vi "读取产品参数信息-CCDA.vi"(8 "错误输入（无错误）":errorcluster, 11 "LoadProductName":string) -> (0 "错误输出":errorcluster)   [LabVIEW 2017]
uses:
  Global System.vi
panel:
  in  "名称或相对路径 2":string="BlackTemplete"
  out "连接的字符串":string
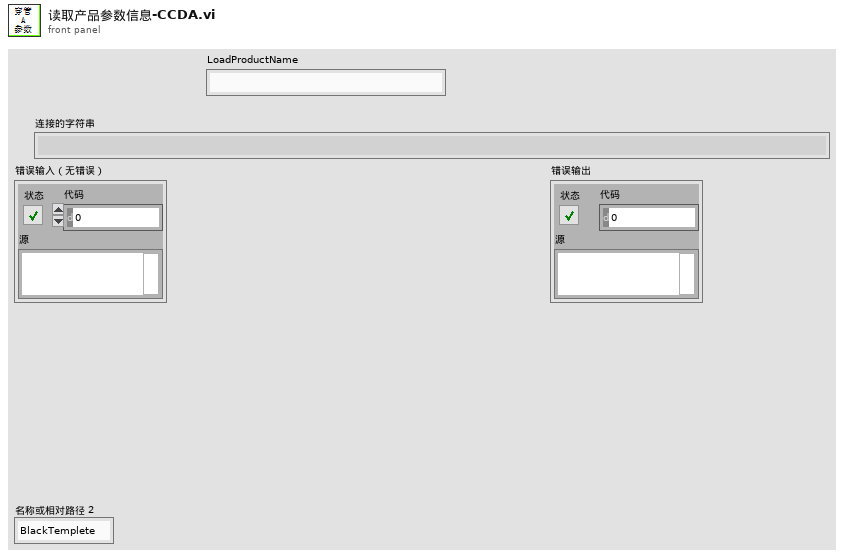
[diagram p1: front panel]
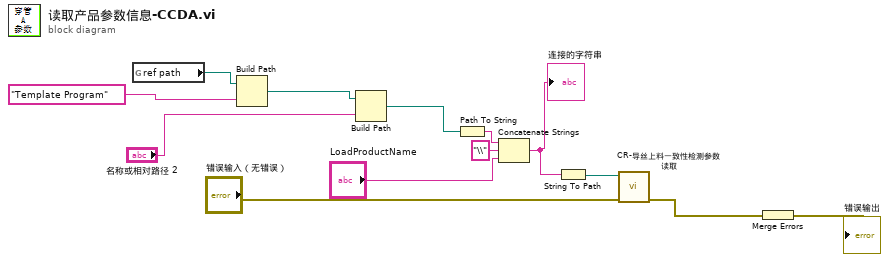
[diagram p0: block diagram]
diagram:
  n1 = global read "Global System.vi" "ref path"() -> (w13:path)
  n2 = Build Path(base path=w13, name or relative path="Template Program" ("名称或相对路径")) -> (appended path=w3:path)
  n3 = Build Path(base path=w3, name or relative path="名称或相对路径 2") -> (appended path=w2:path)
  n4 = Path To String(path=w2) -> (string=w11:string)
  n5 = Concatenate Strings(w11, "\\" ("字符串"), "LoadProductName") -> (w8:string)
  "连接的字符串" <- w8
  n6 = String To Path(string=w8) -> (path=w5:path)
  n7 = call "CR-导丝上料一致性检测参数读取.vi"("error in (no error)"="错误输入（无错误）", "基路径"=w5) -> ("error out"=w7:errorcluster)  [unwired: 5 in, 3 out]
  n8 = Merge Errors(w7) -> (→"错误输出":errorcluster)
